vi "interpolate_color.vi"(9 "Interpolation Value":dbl, 10 "Color2":u32(colorbox), 11 "Color1":u32(colorbox)) -> (3 "Output Color":u32(colorbox))   [LabVIEW 2020, in "3DPC_SurfacePlot.xctl"]
uses:
  <vilib>/Native 3D Graph/xcontrol/3DPC_SurfacePlot.xctl
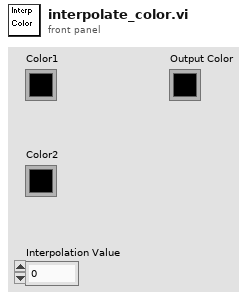
[diagram p1: front panel]
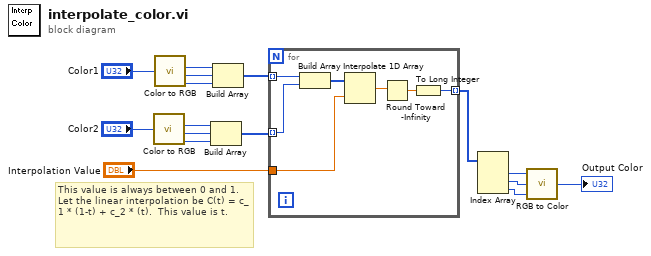
[diagram p0: block diagram]
diagram:
  # "This value is always between 0 and 1.  Let the linear interpolation be C(t) = c_1 * (1-t) + c_2 * (t).  This value is t."
  n1 = call <vilib>:"Color to RGB.vi"("Color"="Color2") -> ("R"=w8:u8, "G"=w9:u8, "B"=w10:u8)  [unwired: 1 out]
  n2 = call <vilib>:"Color to RGB.vi"("Color"="Color1") -> ("R"=w15:u8, "G"=w14:u8, "B"=w13:u8)  [unwired: 1 out]
  n3 = Build Array(w8, w9, w10) -> (w6:u8[])
  n4 = Build Array(w15, w14, w13) -> (w11:u8[])
  n5 = for {
    tunnel: w11 -> [w23] mode=indexing
    tunnel: w6 -> [w22] mode=indexing
    tunnel: "Interpolation Value" -> [w20]
    tunnel: [w17] -> w2 mode=indexing
    n6 = Build Array(w23, w22) -> (w21:u8[])
    n7 = Interpolate 1D Array(1:w20, 2:w21) -> (0:w19:dbl)
    n8 = Round Toward -Infinity(1:w19) -> (0:w18:dbl)
    n9 = To Long Integer(number=w18) -> (32bit integer=w17:i32)
  }
  n10 = Index Array(array=w2) -> (element #1=w5:i32, element #2=w4:i32, element #3=w1:i32)  [unwired: 3 in]
  n11 = call <vilib>:"RGB to Color.vi"("B"=w1, "G"=w4, "R"=w5) -> ("Color"=→"Output Color":u32)
